vi "Delayed Send Async.vi"(6 "Delay ms":i32, 7 "High Priority (F)":bool, 9 "Data":variant, 10 "ID":string, 11 "MessageQ in":refnum<class "MessageQ.lvclass">) -> ()   [LabVIEW 2020, in "Volatus.lvlib" / "MessageQ.lvclass"]
uses:
  MessageQ.lvclass
  MessageQ.lvclass/MessageQ.ctl
  514852db-5662-4e21-bff7-b3befc6de8e5.vi
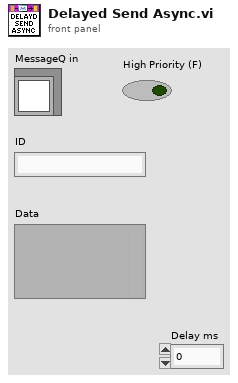
[diagram p1: front panel]
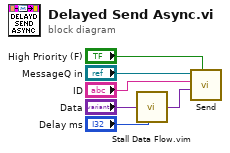
[diagram p0: block diagram]
diagram:
  n1 = call "Stall Data Flow.vim"("value in"="Data", "milliseconds to wait"="Delay ms") -> ("value out"=w2:variant)  [unwired: 1 out]
  n2 = call "Send.vi"("High Priority (F)"="High Priority (F)", "Data"=w2, "ID"="ID", "MessageQ in"="MessageQ in") -> ()  [unwired: 6 in, 2 out]
